vi "Limit Switch Test.vi"() -> ()   [LabVIEW 2025]
uses:
  <vilib>/DAQmx/write.llb/DAQmx Write (Digital 1D Bool 1Chan 1Samp).vi
  <vilib>/DAQmx/read.llb/DAQmx Read (Digital Bool 1Line 1Point).vi
  <vilib>/DAQmx/create/channels.llb/DAQmx Create Channel (DI-Digital Input).vi
  <vilib>/DAQmx/create/channels.llb/DAQmx Create Channel (DO-Digital Output).vi
  <vilib>/DAQmx/miscellaneous.llb/DAQmx Fill In Error Info.vi
  <vilib>/Handler Framework/Handler Framework.lvlib
panel:
  out "error out":errorcluster
  out "data":bool
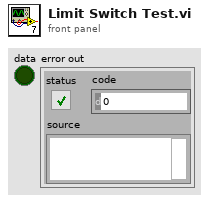
[diagram p1: front panel]
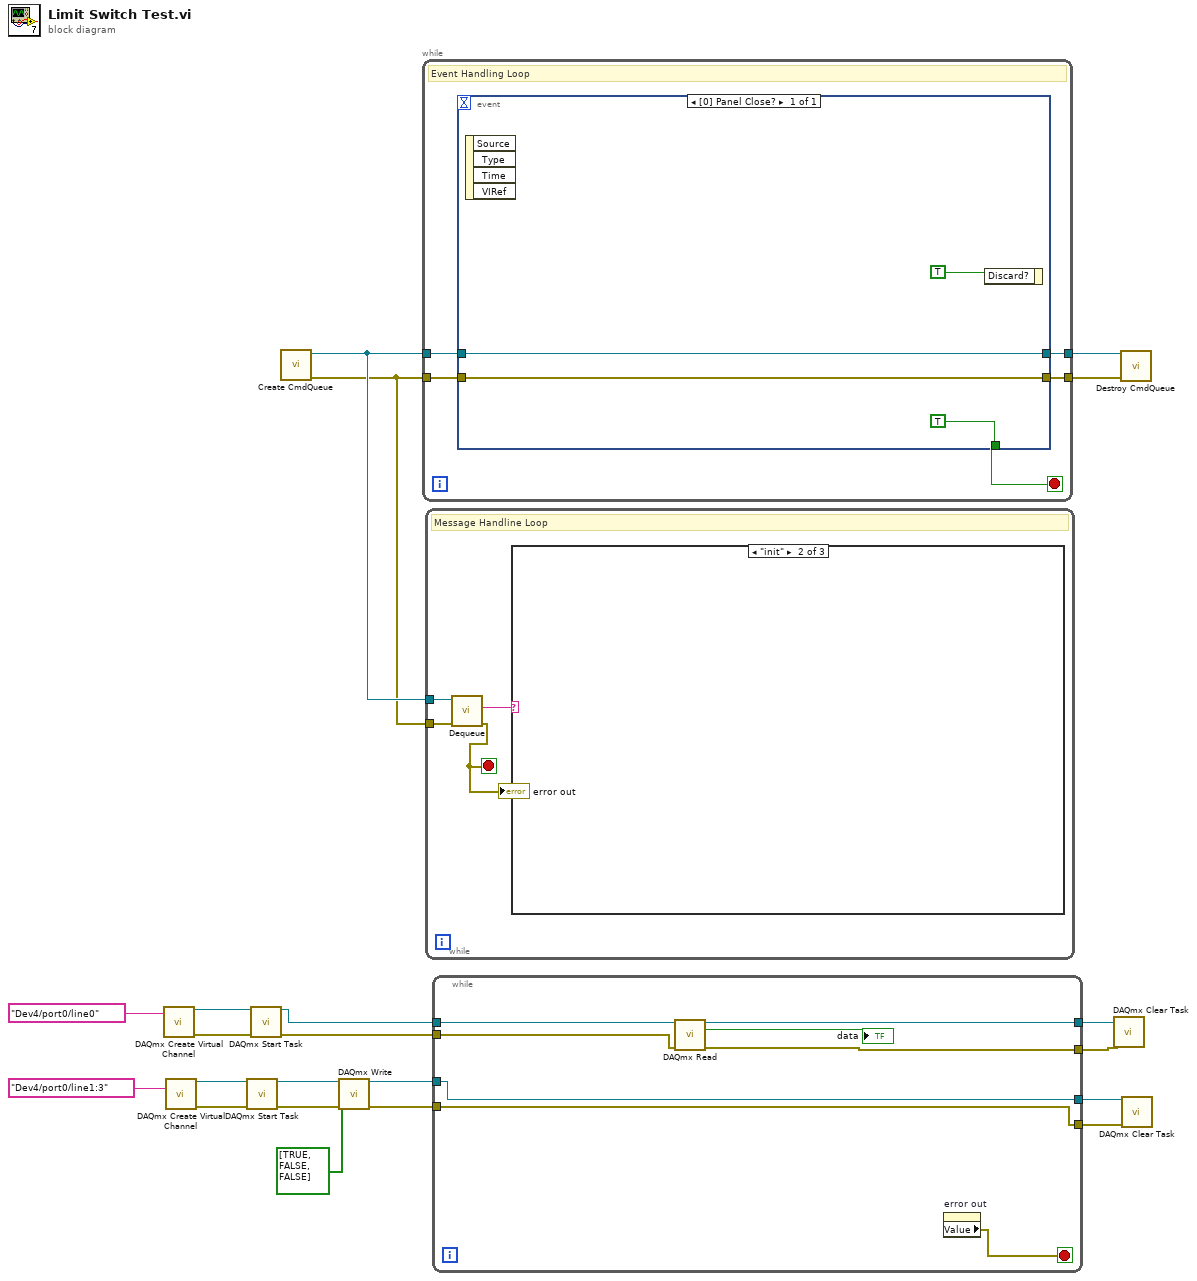
[diagram p0: block diagram]
diagram:
  n1 = call-poly <vilib>:"DAQmx Create Virtual Channel.vi"("lines"=tag "Dev4/port0/line0" ("physical channels")) -> ("task out"=w15:refnum<k21>, "error out"=w14:errorcluster)  [unwired: 13 in]
  n2 = call-poly <vilib>:"DAQmx Create Virtual Channel.vi"("lines"=tag "Dev4/port0/line1:3") -> ("task out"=w13:refnum<k21>, "error out"=w12:errorcluster)  [unwired: 13 in]
  n3 = call <vilib>:"DAQmx Start Task.vi"("task/channels in"=w13, "error in"=w12) -> ("task out"=w11:refnum<k21>, "error out"=w10:errorcluster)  [unwired: 12 in]
  n4 = call <vilib>:"DAQmx Start Task.vi"("task/channels in"=w15, "error in"=w14) -> ("task out"=w9:refnum<k21>, "error out"=w8:errorcluster)  [unwired: 12 in]
  n5 = call <vilib>:"Create CmdQueue.vi"() -> ("error out"=w20:errorcluster, "CmdQueue out"=w21:refnum<queue>)  [unwired: 10 in]
  n6 = call-poly <vilib>:"DAQmx Write.vi"("task/channels in"=w11, "data"=bool[] [TRUE, FALSE, FALSE], "error in"=w10) -> ("task out"=w3:refnum<k21>, "error out"=w4:errorcluster)  [unwired: 10 in, 1 out]
  n7 = while {
    tunnel: w21 -> [w25]
    tunnel: w20 -> [w24]
    tunnel: [w23] -> w19
    tunnel: [w22] -> w18
    stop <- w26 stop-if-true
    # "Event Handling Loop"
    n8 = event shown="[0] Panel Close?" {
      selector: _ -> [_]
      dyn-events: _ -> [_]
      timeout: _ -> [_]
      tunnel: [TRUE] -> w26
      tunnel: w25 -> [w28]
      tunnel: w24 -> [w27]
      tunnel: [w28] -> w23
      tunnel: [w27] -> w22
      event Panel Close? {
        n9 = event-data() -> ()  [unwired: 1 in, 4 out]
        n10 = event-data("Discard?"=TRUE) -> ()  [unwired: 1 in, 1 out]
      }
    }
  }
  n11 = while {
    tunnel: w21 -> [w34]
    tunnel: w20 -> [w33]
    stop <- w32 stop-if-true
    # "Message Handline Loop"
    n12 = call <vilib>:"Dequeue.vi"("error in (no error)"=w33, "CmdQueue in"=w34) -> ("error out"=w32:errorcluster, "cmd"=w31:string)  [unwired: 5 in, 3 out]
    "error out" <- w32
    n13 = case shown="\"init\"" w31 {
      frame Default {
      }
      frame "init" {
      }
      frame "shutdown" {
      }
    }
  }
  n14 = while {
    tunnel: w9 -> [w42]
    tunnel: w8 -> [w41]
    tunnel: [w39] -> w7
    tunnel: [w38] -> w6
    tunnel: [w37] -> w5
    tunnel: w4 -> [w37]
    tunnel: w3 -> [w36]
    tunnel: [w36] -> w2
    stop <- w35 stop-if-true
    n15 = call-poly <vilib>:"DAQmx Read.vi"("task/channels in"=w42, "error in"=w41) -> ("task out"=w39:refnum<k21>, "data"=→"data":bool, "error out"=w38:errorcluster)  [unwired: 11 in]
    n16 = property on="error out" class="Clust (strict)"() -> ("Value"=w35:errorcluster)  [unwired: 2 in, 2 out]
  }
  n17 = call <vilib>:"DAQmx Clear Task.vi"("task in"=w7, "error in"=w6) -> ()  [unwired: 13 in, 1 out]
  n18 = call <vilib>:"Destroy CmdQueue.vi"("error in (no error)"=w18, "CmdQueue in"=w19) -> ()  [unwired: 9 in, 1 out]
  n19 = call <vilib>:"DAQmx Clear Task.vi"("task in"=w2, "error in"=w5) -> ()  [unwired: 13 in, 1 out]
